vi "sample moves.vi"(4 "move time":dbl[unit], 6 "current time":dbl[unit] format="%<%H:%M:%S%2u>t", 7 "Gilson ID":i32, 8 "initialize":bool, 9 "vial position":T1, 10 "Samples":T4, 11 "sample ID":i16) -> (2 "sampler state":T3, 3 "sample ID out":i16)   [LabVIEW 2012]
uses:
  sampler states.ctl
  Samples.ctl
  point.ctl
  vial position.ctl
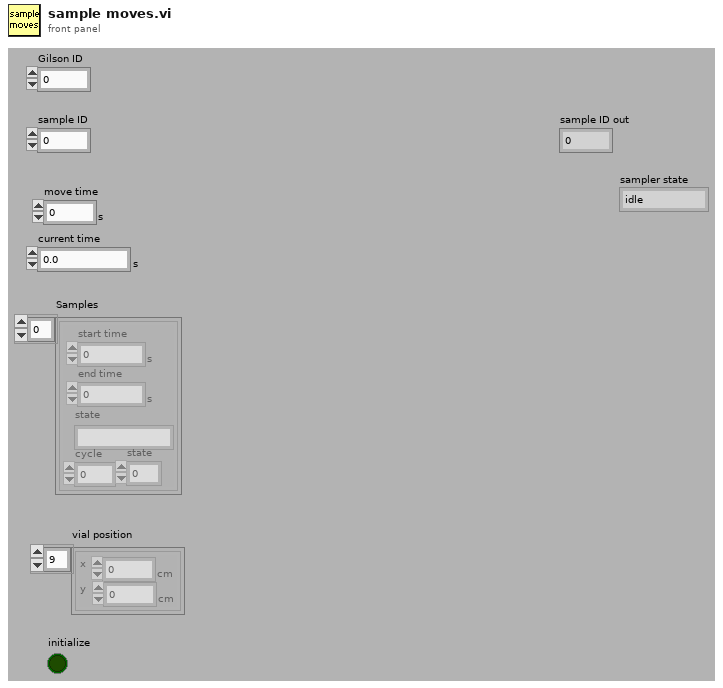
[diagram p1: front panel]
types:
  T1 = typedef "vial position.ctl" = T2[]
  T2 = typedef "point.ctl" = cluster{"x":dbl[unit], "y":dbl[unit]}
  T3 = typedef "sampler states.ctl" = enum16{"idle", "go sample loc", "collect sample", "go home"}
  T4 = typedef "Samples.ctl" = cluster{"start time":dbl[unit], "end time":dbl[unit], "state":string, "cycle":u16, "state":u16}[]
  T5 = cluster{"start time":dbl[unit], "end time":dbl[unit], "state":string, "cycle":u16, "state":u16}
  T6 = enum16{"idle", "go sample loc", "collect sample", "go home"}
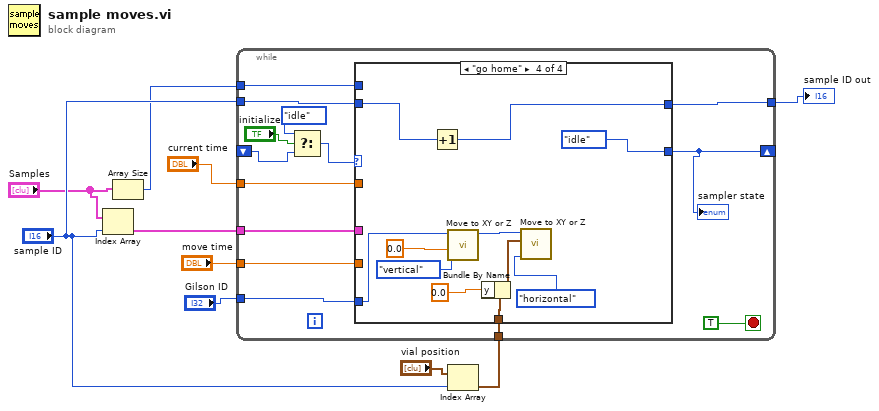
[diagram p0: block diagram]
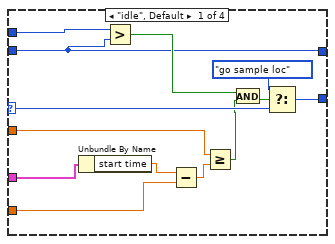
[diagram p2: hidden frame]
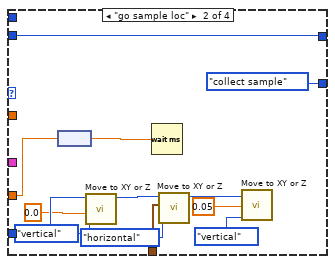
[diagram p3: hidden frame]
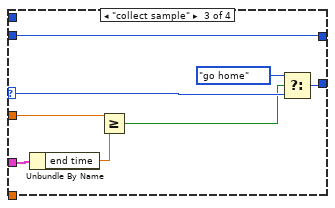
[diagram p4: hidden frame]
diagram:
  n1 = Index Array(array="Samples", index="sample ID") -> (element=w10:T5)
  n2 = Array Size(array="Samples") -> (size(s)=w1:i32)
  n3 = Index Array(array="vial position", index="sample ID") -> (element=w6:T2)
  n4 = while {
    shift-right: [w24] -> _
    shift-left: _ -> [w15]
    tunnel: w10 -> [w23]
    tunnel: "current time" -> [w22]
    tunnel: "Gilson ID" -> [w21]
    tunnel: w6 -> [w20]
    tunnel: "move time" -> [w19]
    tunnel: "sample ID" -> [w17]
    tunnel: [w16] -> w3
    tunnel: w1 -> [w11]
    stop <- TRUE stop-if-true
    n5 = Select(t=T6."idle", s="initialize", f=w15) -> (s? t:f=w14:T3)
    n6 = case shown="\"go home\"" w14 {
      selector: w14 -> [w37 _ w58 _]
      tunnel: [w36 sampler_states."collect sample" ("t") w57 sampler_states."idle" ("t")] -> w24
      tunnel: w23 -> [w34 _ w55 _]
      tunnel: w22 -> [w31 _ w54 _]
      tunnel: w21 -> [_ w50 _ w66]
      tunnel: w20 -> [_ w48 _ w64]
      tunnel: w19 -> [w30 w44 _ _]
      tunnel: w17 -> [w25 w38 w51 w60]
      tunnel: [w25 w38 w51 w59] -> w16
      tunnel: w11 -> [w29 _ _ _]
      frame "idle", Default {
        n7 = Unbundle By Name(w34) -> ("start time"=w33:dbl[unit])
        n8 = Greater?(x=w29, y=w25) -> (0:w28:bool)
        n9 = Subtract(x=w33, y=w30) -> (x-y=w32:dbl[unit])
        n10 = Greater Or Equal?(x=w31, y=w32) -> (x >= y?=w27:bool)
        n11 = And(x=w28, y=w27) -> (x .and. y?=w26:bool)
        n12 = Select(t=sampler_states."go sample loc", s=w26, f=w37) -> (s? t:f=w36:T3)
      }
      frame "go sample loc" {
        n13 = node(w44) -> (w43:dbl)
        n14 = call "Move to XY or Z.vi"("move type"=enum16{"horizontal", "vertical"}."vertical", "Z"=dbl[unit] 0.0, "ID"=w50) -> ("ID out"=w49:i32)  [unwired: 7 in, 1 out]
        n15 = Wait (ms)(milliseconds to wait=w43) -> ()  [unwired: 1 out]
        n16 = call "Move to XY or Z.vi"("move type"=enum16{"horizontal", "vertical"}."horizontal", "position 1"=w48, "ID"=w49) -> ("ID out"=w41:i32)  [unwired: 7 in, 1 out]
        n17 = call "Move to XY or Z.vi"("move type"=enum16{"horizontal", "vertical"}."vertical", "Z"=dbl[unit] 0.05, "ID"=w41) -> ()  [unwired: 7 in, 2 out]
      }
      frame "collect sample" {
        n18 = Unbundle By Name(w55) -> ("end time"=w53:dbl[unit])
        n19 = Greater Or Equal?(x=w54, y=w53) -> (x >= y?=w52:bool)
        n20 = Select(t=sampler_states."go home", s=w52, f=w58) -> (s? t:f=w57:T3)
      }
      frame "go home" {
        n21 = Increment(x=w60) -> (x+1=w59:i16)
        n22 = call "Move to XY or Z.vi"("move type"=enum16{"horizontal", "vertical"}."vertical", "Z"=dbl[unit] 0.0, "ID"=w66) -> ("ID out"=w69:i32)  [unwired: 7 in, 1 out]
        n23 = Bundle By Name(cluster=w64, "y"=dbl[unit] 0.0) -> (w62:T2)
        n24 = call "Move to XY or Z.vi"("move type"=enum16{"horizontal", "vertical"}."horizontal", "position 1"=w62, "ID"=w69) -> ()  [unwired: 7 in, 2 out]
      }
    }
    "sampler state" <- w24
  }
  "sample ID out" <- w3
